vi "Configure Settings.vi"   [LabVIEW 2017]
uses:
  acquisition/Acquisition Settings.ctl
  acquisition/Acquisition State.ctl
  logging/Logging Configuration.ctl
  logging/Logging State.ctl
  support/libs/PMU Buffer/Buffer Settings.ctl
  processing/Processing Settings.ctl
  processing/BP Filter Settings.ctl
  <vilib>/Analysis/3filter.llb/Filter Passband Type.ctl
  support/libs/Signal Selector/Selection Folder/Signal types.ctl
  processing/Levels.ctl
  processing/Filters.ctl
  processing/PSD Setting.ctl
  2a34ae97-60f5-4341-84c9-4d8c7df74f18.vi
  3968f581-f6d6-4989-85de-0e430d724e00.vi
  38842cf4-451f-4579-bb41-44dc6a1ccd67.vi
  8eb40251-70cd-4357-b466-147393c2f03b.vi
  a47746fd-76d0-4c2d-aaac-f7d470606d9a.vi
  290ce276-0645-466b-8e97-8b13ac2f5f93.vi
  support/settings/Get Config File Path.vi
  <vilib>/Utility/xml.llb/Read From XML File.vi
  <vilib>/Utility/xml.llb/Read From XML File(string).vi
  <vilib>/Utility/xml.llb/Write to XML File.vi
  <vilib>/Utility/xml.llb/Write to XML File(string).vi
  acquisition/Acquisition.lvlib
  support/libs/PMU Buffer/PMU data buffer.lvlib
  logging/Logging.lvlib
  processing/Processing.lvlib
  support/libs/Signal Selector/Selection Folder/Selection.xctl
  <vilib>/Analysis/NI_AALBase.lvlib
  support/settings/Settings Dialog.vi
  support/settings/Settings.lvlib
panel:
  # "RUN this VI to load the current settings into the settings dialog, edit them and save them on disk"
types:
  T1 = typedef "Processing.lvlib/Processing Settings.ctl" = cluster{"Settings":string, "Refresh Rate":u32, "Filter Config":T2[], "Params Energy":T4, "Selection Energy":cluster{"Type":T5, "Index(es)":i32[]}[], "Levels":T6, "Filters Instances":T7[], "PSDs":refnum<vi>[], "Params PSD":T4, "Signal PSD":cluster{"Type":T5, "Index(es)":i32[]}[], "PSD Instances":T8[]}
  T2 = typedef "Processing.lvlib/BP Filter Settings.ctl" = cluster{"Type":T3, "Freq low":dbl, "Freq high":dbl, "Order":i32}
  T3 = typedef "NI_AALBase.lvlib/Filter Passband Type.ctl" = enum32{"Lowpass", "Highpass", "Bandpass", "Bandstop"}
  T4 = typedef "PMU data buffer.lvlib/Buffer Settings.ctl" = cluster{"Index":i32, "Size":i32, "Samples":i32, "Ordered ?":bool}
  T5 = typedef "Selection.xctl/Signal types.ctl" = enum16{"Disable", "Frequency", "Phasor Mag", "Phasor Ang", "Angle Diff"}
  T6 = typedef "Processing.lvlib/Levels.ctl" = cluster{"Low":i32, "High":i32, "Danger":i32}
  T7 = typedef "Processing.lvlib/Filters.ctl" = cluster{"BP Filter":dbl[], "Delay":dbl[], "MA Filter":dbl[], "PSD Filter":cluster{"filter structure":enum32{"IIR 2nd Order", "IIR 4th Order"}, "Reverse Coefficients":dbl[], "Forward Coefficients":dbl[]}, "Decimation":i32}
  T8 = typedef "Processing.lvlib/PSD Setting.ctl" = cluster{"dB on? (T)":bool, "Reset":bool, "AR":cluster{"Bins":i32, "AR order":i32, "Method":u16}, "Welch":cluster{"window info":cluster{"window":u16, "length":i32, "overlap (%)":dbl}, "Bins":i32}, "Method":enum16{"Method Welch", "Method AR", "Both"}, "Averaging":cluster{"averaging mode":u16, "weighting mode":u16, "number of averages":u32}}
  T9 = typedef "Logging.lvlib/Logging Configuration.ctl" = cluster{"Logging State":T10, "Settings":string, "Buffer":T4}
  T10 = typedef "Logging.lvlib/Logging State.ctl" = enum16{"Idle", "Logging"}
  T11 = typedef "Acquisition.lvlib/Acquisition Settings.ctl" = cluster{"State":T12, "Settings":string, "Online":bool, "S3DK":cluster{"Signals":cluster{"Phasor":string[], "Analog":string[], "Digital":string[]}}, "CSV":cluster{"CSV Path":path, "Index":i32, "Parcel Length":i32, "EOF?":bool}}
  T12 = typedef "Acquisition.lvlib/Acquisition State.ctl" = enum16{"Idle", "Idle S3DK", "Acquiring S3DK", "Idle CSV", "Acquiring CSV"}
  T13 = cluster{"Settings Out":T11, "Settings Out":T9, "Settings Out":T1}
  T14 = typedef "Settings.lvlib/Settings.ctl" = cluster{"Acquisition":T11, "Logging":T9, "Processing":T1}
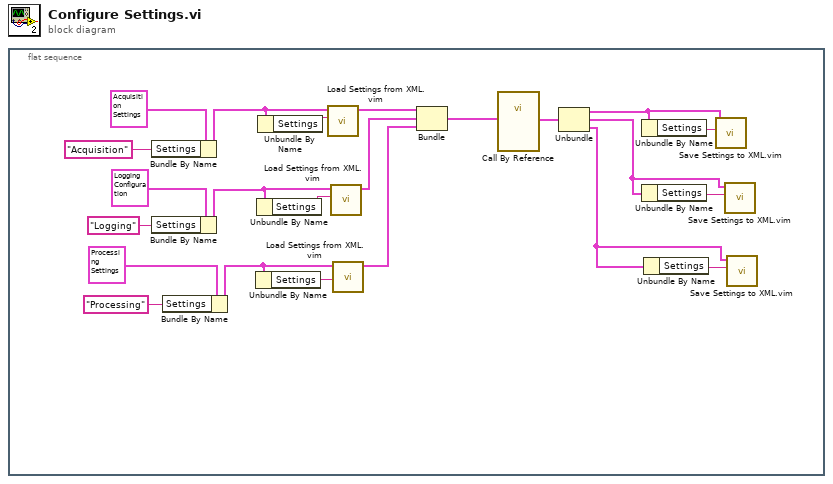
[diagram p0: block diagram]
diagram:
  n1 = flat-sequence {
    frame #0 {
      n2 = Bundle By Name(cluster=T11 {"State"=enum."Idle S3DK", "Settings"="Acquisition", "Online"=FALSE, "S3DK"={"Signals"={"Phasor"=[], "Analog"=[], "Digital"=[]}}, "CSV"={"CSV Path"=path "", "Index"=0, "Parcel Length"=0, "EOF?"=FALSE}} ("Data Cluster"), "Settings"="Acquisition") -> (w17:T11)
      n3 = Bundle By Name(cluster=T9 {"Logging State"=enum."Idle", "Settings"="Logging", "Buffer"={"Index"=0, "Size"=15000, "Samples"=0, "Ordered ?"=FALSE}} ("Logging Configuration"), "Settings"="Logging") -> (w15:T9)
      n4 = Bundle By Name(cluster=T1 {"Settings"="Processing", "Refresh Rate"=0, "Filter Config"=[], "Params Energy"={"Index"=0, "Size"=0, "Samples"=0, "Ordered ?"=FALSE}, "Selection Energy"=[], "Levels"={"Low"=0, "High"=0, "Danger"=0}, "Filters Instances"=[], "PSDs"=[], "Params PSD"={"Index"=0, "Size"=0, "Samples"=0, "Ordered ?"=FALSE}, "Signal PSD"=[], "PSD Instances"=[]} ("Processing Settings"), "Settings"="Processing") -> (w13:T1)
      n5 = Unbundle By Name(w13) -> ("Settings"=w12:string)
      n6 = Unbundle By Name(w15) -> ("Settings"=w14:string)
      n7 = Unbundle By Name(w17) -> ("Settings"=w16:string)
      n8 = call "Load Settings from XML.vim"("Settings File Name"=w16, "Settings In"=w17) -> ("Settings Out"=w11:T11)  [unwired: 8 in, 1 out]
      n9 = call "Load Settings from XML.vim"("Settings File Name"=w14, "Settings In"=w15) -> ("Settings Out"=w10:T9)  [unwired: 8 in, 1 out]
      n10 = call "Load Settings from XML.vim"("Settings File Name"=w12, "Settings In"=w13) -> ("Settings Out"=w9:T1)  [unwired: 8 in, 1 out]
      n11 = Bundle("Settings Out"=w11, "Settings Out"=w10, "Settings Out"=w9) -> (w8:T13)  [unwired: 1 in]
      n12 = call-by-ref "?"("Settings in"=w8) -> ("Settings out"=w6:T14)  [unwired: 9 in, 5 out]
      n13 = Unbundle(w6) -> ("Acquisition"=w3:T11, "Logging"=w2:T9, "Processing"=w1:T1)
      n14 = Unbundle By Name(w3) -> ("Settings"=w7:string)
      n15 = Unbundle By Name(w2) -> ("Settings"=w5:string)
      n16 = Unbundle By Name(w1) -> ("Settings"=w4:string)
      n17 = call "Save Settings to XML.vim"("Settings File Name"=w7, "Settings In"=w3) -> ()  [unwired: 9 in, 1 out]
      n18 = call "Save Settings to XML.vim"("Settings File Name"=w5, "Settings In"=w2) -> ()  [unwired: 9 in, 1 out]
      n19 = call "Save Settings to XML.vim"("Settings File Name"=w4, "Settings In"=w1) -> ()  [unwired: 9 in, 1 out]
    }
  }
